vi "Odour_chemicals.vi"() -> (0 "Odour chemicals":T1(array[cluster]))   [LabVIEW 2016]
uses:
  <vilib>/Utility/file.llb/Read Delimited Spreadsheet (string).vi
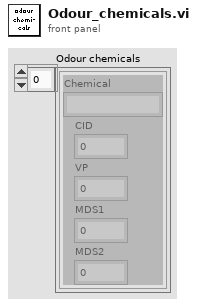
[diagram p1: front panel]
types:
  T1 = cluster{"Chemical":string, "CID":i32, "VP":dbl, "MDS1":dbl, "MDS2":dbl}[]
  T2 = cluster{"Chemical":string, "CID":i32, "VP":dbl, "MDS1":dbl, "MDS2":dbl}
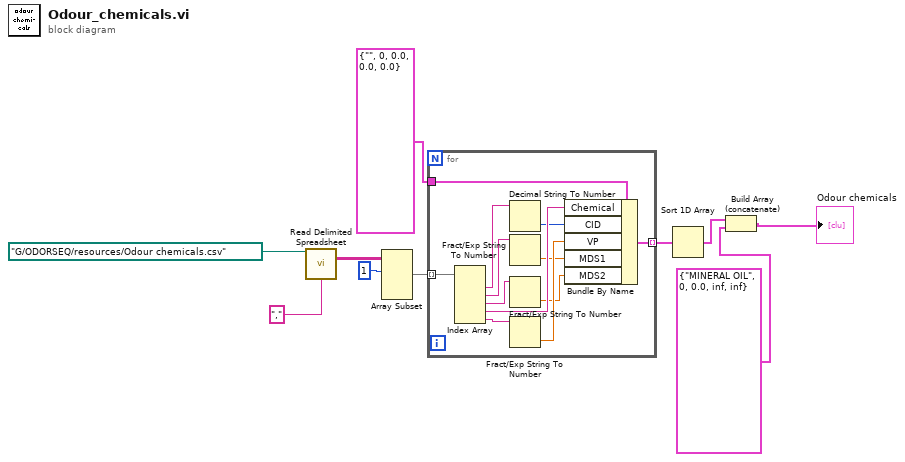
[diagram p0: block diagram]
diagram:
  n1 = call-poly <vilib>:"Read Delimited Spreadsheet.vi"("file path (dialog if empty)"=path "G:/ODORSEQ/resources/Odour chemicals.csv", "delimiter (\\t)"="," ("delimiter (\\t)")) -> ("all rows"=w9:string[][])  [unwired: 8 in, 5 out]
  n2 = Array Subset(array=w9, index (row)=1 ("index")) -> (w10:string[][])  [unwired: 3 in]
  n3 = for {
    tunnel: w10 -> [w21] mode=indexing
    tunnel: T2 {"Chemical"="", "CID"=0, "VP"=0.0, "MDS1"=0.0, "MDS2"=0.0} ("input cluster") -> [w22]
    tunnel: [w20] -> w4 mode=indexing
    n4 = Index Array(array=w21) -> (element #1=w16:string, element #2=w14:string, element #3=w12:string, element #4=w19:string, element #5=w18:string)  [unwired: 5 in]
    n5 = Decimal String To Number(string=w16) -> (number=w15:i32)  [unwired: 2 in, 1 out]
    n6 = Fract/Exp String To Number(string=w14) -> (number=w13:dbl)  [unwired: 3 in, 1 out]
    n7 = Fract/Exp String To Number(string=w12) -> (number=w11:dbl)  [unwired: 3 in, 1 out]
    n8 = Fract/Exp String To Number(string=w18) -> (number=w17:dbl)  [unwired: 3 in, 1 out]
    n9 = Bundle By Name(cluster=w22, "Chemical"=w19, "CID"=w15, "VP"=w17, "MDS1"=w13, "MDS2"=w11) -> (w20:T2)
  }
  n10 = Sort 1D Array(array=w4) -> (sorted array=w2:T1)
  n11 = Build Array (concatenate)(w2, T2 {"Chemical"="MINERAL OIL", "CID"=0, "VP"=0.0, "MDS1"=inf, "MDS2"=inf} ("input cluster")) -> (→"Odour chemicals":T1)
